vi "Set Oscillator Frequency Sweep Stop Frequency.vi"(8 "error in (no error)":errorcluster, 10 "Oscillator Frequency Sweep Stop Frequency (Hz)":dbl min=0.0 max=250000.0 step=0.001, 11 "SR7270 Drivers in":refnum<class "SR7270 Drivers.lvclass">) -> (0 "error out":errorcluster, 3 "SR7270 Drivers out":refnum<class "SR7270 Drivers.lvclass">)   [LabVIEW 2016, in "SR7270 Drivers.lvclass"]
uses:
  SR7270 Drivers.lvclass
  SR7270 Drivers.lvclass/SR7270 Drivers.ctl
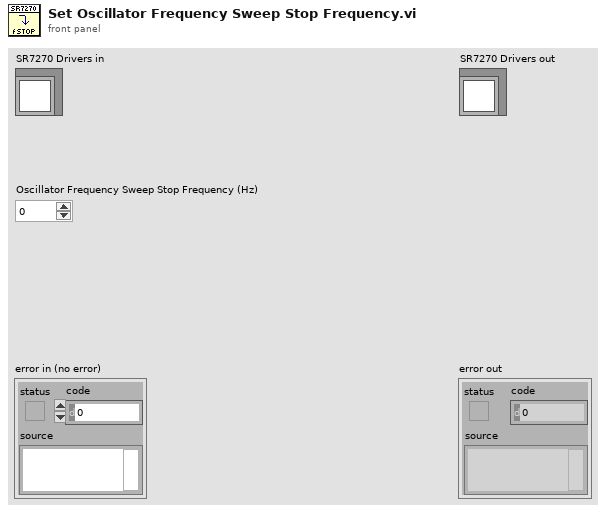
[diagram p1: front panel]
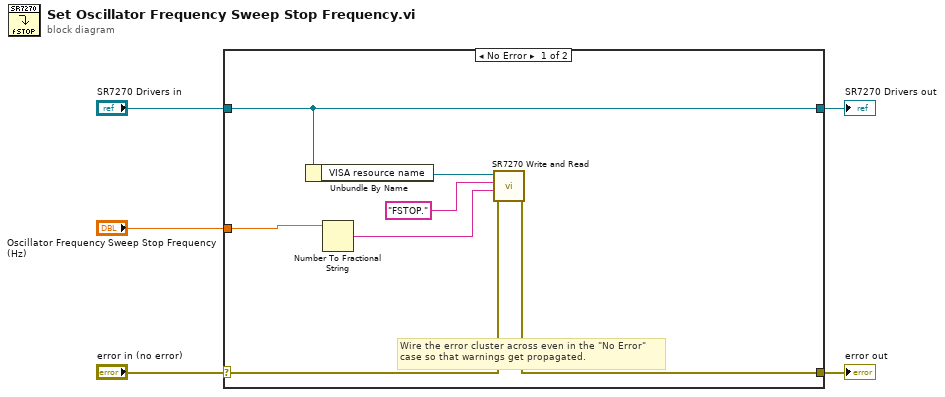
[diagram p0: block diagram]
diagram:
  n1 = case shown="No Error" "error in (no error)" {
    selector: "error in (no error)" -> [w10 w14]
    tunnel: [w9 w14] -> w4
    tunnel: [w11 w13] -> w2
    tunnel: "SR7270 Drivers in" -> [w11 w13]
    tunnel: "Oscillator Frequency Sweep Stop Frequency (Hz)" -> [w8 _]
    frame No Error {
      # "Wire the error cluster across even in the \"No Error\"\ncase so that warnings get propagated."
      n2 = Unbundle By Name(w11) -> ("VISA resource name"=w12:refnum<visa-resource-name>)
      n3 = Number To Fractional String(number=w8) -> (F-format string=w6:string)  [unwired: 3 in]
      n4 = call "SR7270 Write and Read.vi"("error in (no error)"=w10, "Parameter(s)"=w6, "Command Name"="FSTOP.", "VISA resource name"=w12) -> ("error out"=w9:errorcluster)  [unwired: 4 in, 3 out]
    }
    frame Error {
    }
  }
  "error out" <- w4
  "SR7270 Drivers out" <- w2
